vi "DSP Configure.vi"(8 "error in":errorcluster, 9 "duration [s]":dbl=0.1, 10 "Rate [Hz]":dbl, 11 "MicroDAQ.lvlib:DSP.lvclass":refnum<class "DSP.lvclass">) -> (0 "error out":errorcluster, 3 "MicroDAQ.lvlib:DSP.lvclass out":refnum<class "DSP.lvclass">)   [LabVIEW 2009, in "MicroDAQ.lvlib" / "DSP.lvclass"]
doc: "This VI configre DSP task and loads it to device. Its must be done before DSP start function is run."
uses:
  <instrlib>/MicroDAQ/Channel/DSP/DSP.lvclass
  <instrlib>/MicroDAQ/Channel/DSP/DSP.lvclass/DSP.ctl
  <instrlib>/MicroDAQ/Mlink library wraper/mlink.lvlib
  <instrlib>/MicroDAQ/Channel/Channel.lvclass
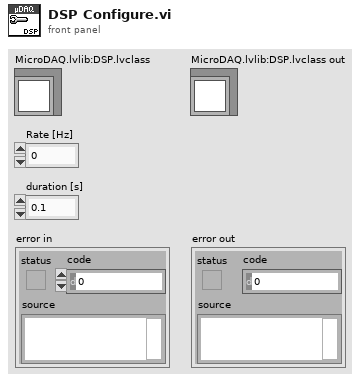
[diagram p1: front panel]
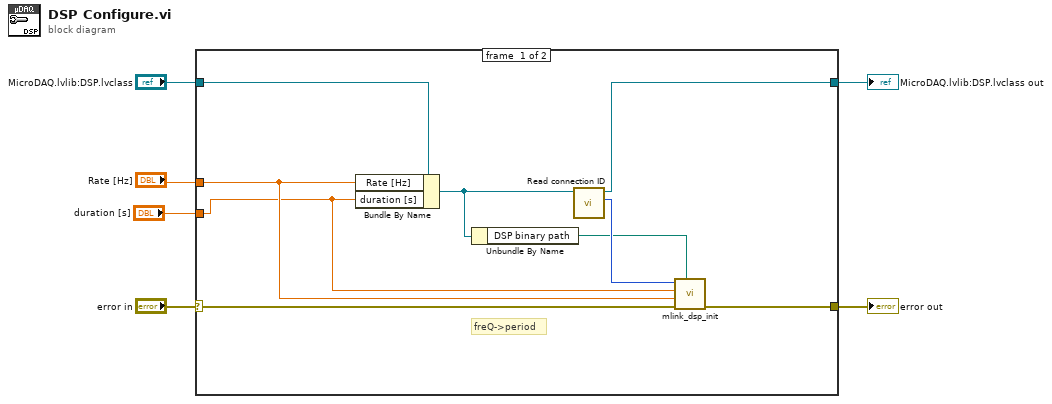
[diagram p0: block diagram]
diagram:
  n1 = case shown="No Error" "error in" {
    selector: "error in" -> [w14 w16]
    tunnel: "MicroDAQ.lvlib:DSP.lvclass" -> [w15 w17]
    tunnel: [w13 w16] -> w5
    tunnel: [w12 w17] -> w3
    tunnel: "Rate [Hz]" -> [w9 _]
    tunnel: "duration [s]" -> [w8 _]
    frame #0 {
      # "freQ->period"
      n2 = Bundle By Name(cluster=w15, "Rate [Hz]"=w9, "duration [s]"=w8) -> (w10:refnum<class "DSP.lvclass">)
      n3 = Unbundle By Name(w10) -> ("DSP binary path"=w7:path)
      n4 = call <instrlib>:"Read connection ID.vi"("Task in"=w10) -> ("connection ID"=w11:i32, "Task out"=w12:refnum<class "DSP.lvclass">)  [unwired: 9 in]
      n5 = call <instrlib>:"mlink_dsp_init.vi"("DSP binary path"=w7, "error in (no error)"=w14, "rate [period s]"=w9, "duration [s]"=w8, "connection ID"=w11) -> ("error out"=w13:errorcluster)  [unwired: 5 in, 1 out]
    }
    frame #1 {
    }
  }
  "error out" <- w5
  "MicroDAQ.lvlib:DSP.lvclass out" <- w3
